vi "USB-6008-AnalogIn.vi"() -> ()   [LabVIEW 2010]
panel:
  out "Array of Waveform":waveform(dbl)[](array[waveform])
  out "Waveform Chart":waveform(dbl)[](graph)
  in  "number of samples":i32=1000
  in  "rate":dbl=1000.0
  in  "stop":bool
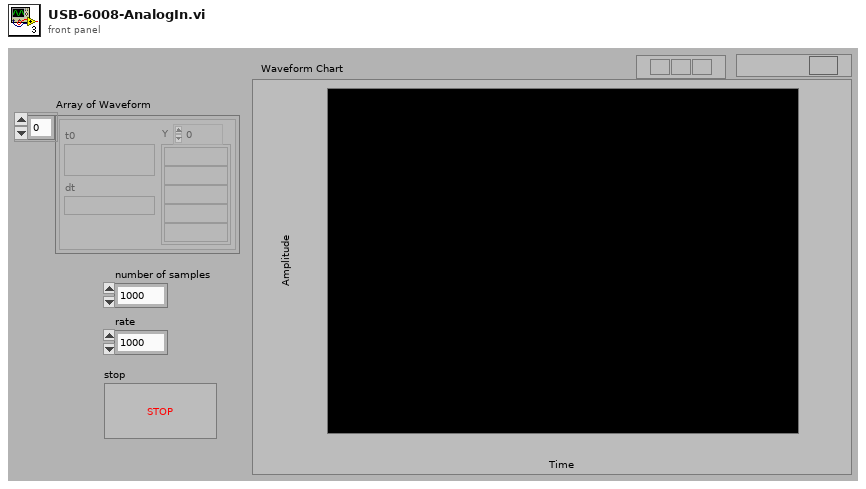
[diagram p1: front panel]
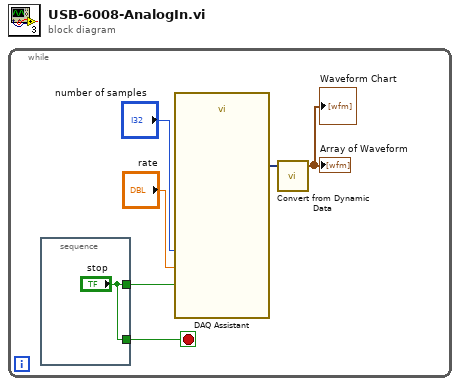
[diagram p0: block diagram]
diagram:
  n1 = while "WhileLoop" {
    stop <- w6 stop-if-true
    n2 = stacked-sequence {
      tunnel: ["stop"] -> w5
      tunnel: ["stop"] -> w6
      frame #0 {
      }
    }
    n3 = call "DAQ Assistant"("rate"="rate", "number of samples"="number of samples", "stop (F)"=w5) -> ("data"=w4:dynamicdata)  [unwired: 13 in, 3 out]
    n4 = call "Convert from Dynamic Data"("Dynamic Data Type"=w4) -> ("Array of Waveform"=→"Waveform Chart" →"Array of Waveform":waveform(dbl)[])  [unwired: 3 in]
  }
